vi "has_repeated_capability_solution.vi"(8 "error in (no error)":errorcluster, 11 "Instrument Command In":string) -> (0 "error out":errorcluster, 3 "Instrument Command Out":string)   [LabVIEW 2018]
uses:
  <vilib>/regexp/Match Regular Expression.xnode
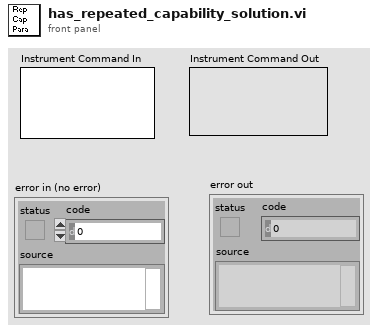
[diagram p1: front panel]
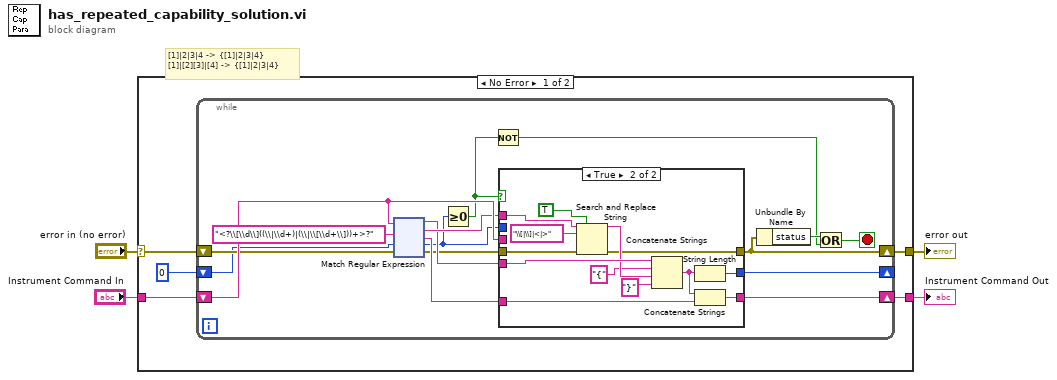
[diagram p0: block diagram]
diagram:
  # "[1]|2|3|4 -> {[1]|2|3|4}\n[1]|[2][3]|[4] -> {[1]|2|3|4}"
  n1 = case shown="No Error" "error in (no error)" {
    selector: "error in (no error)" -> [w6 w153]
    tunnel: [w9 w154] -> w4
    tunnel: "Instrument Command In" -> [w8 w154]
    tunnel: [w5 w153] -> w1
    frame No Error {
      n2 = while {
        shift-right: [w25] -> w9
        shift-left: w8 -> [w24]
        shift-right: [w11] -> _
        shift-left: 0 ("offset past match") -> [w12]
        shift-right: [w19] -> w5
        shift-left: w6 -> [w23]
        stop <- w20 stop-if-true
        n3 = xnode "Match Regular Expression"("input string"=w24, "regular expression"="<?\\[\\d\\]((\\|\\d+)|(\\|\\[\\d+\\]))+>?", "offset (0)"=w12, "error in"=w23) -> ("before match"=w16:string, "whole match"=w17:string, "after match"=w15:string, "offset past match"=w10:i32, "error out"=w13:errorcluster)  [unwired: 2 out]
        n4 = Greater Or Equal To 0?(x=w10) -> (x >= 0?=w14:bool)
        n5 = Not(x=w14) -> (.not. x?=w21:bool)
        n6 = case shown="True" w14 {
          tunnel: w17 -> [_ w40]
          tunnel: w16 -> [_ w41]
          tunnel: w15 -> [_ w32]
          tunnel: [w28 w31] -> w25
          tunnel: w24 -> [w28 _]
          tunnel: w13 -> [w27 w34]
          tunnel: [w27 w33] -> w19
          tunnel: [w26 w29] -> w11
          tunnel: w10 -> [w26 _]
          frame False {
          }
          frame True {
            n7 = Search and Replace String(replace all?=TRUE ("replace all? (F)"), input string=w40, search string="\\[|\\]|<|>", error in=w34) -> (result string=w37:string, error out=w33:errorcluster)  [unwired: 6 out]
            n8 = Concatenate Strings(w41, "{" ("string"), w37, "}" ("string")) -> (w30:string)
            n9 = String Length(string=w30) -> (length=w29:i32)
            n10 = Concatenate Strings(w30, w32) -> (w31:string)
          }
        }
        n11 = Unbundle By Name(w19) -> ("status"=w22:bool)
        n12 = Or(x=w22, y=w21) -> (x .or. y?=w20:bool)
      }
    }
    frame Error {
    }
  }
  "Instrument Command Out" <- w4
  "error out" <- w1
